vi "analoginput_software_trigger_daqmxbasemodified.vi"() -> ()   [LabVIEW 2014]
doc: "This VI compares analog data from a DAQ device in software to some trigger level. Once the condition is met the VI in software initiates a digital right to a pin on a DAQ device."
uses:
  <vilib>/_DAQmxBase/Internals/DAQmxBase Read (Analog 1D DBL NChan 1Samp).vi
  <vilib>/_DAQmxBase/Internals/DAQmxBase Timing (Sample Clock).vi
  <vilib>/_DAQmxBase/Internals/DAQmxBase Create Channel (AI-Voltage-Basic).vi
panel:
  in  "Analog Clock Source":tag
  in  "Analog Channel":tag="Dev1/ai0"
  in  "Analog Sample Mode":T1(ring)=enum."Hardware Timed Single Point"
  in  "Sample Rate":dbl=1000.0 format="%#_13g"
  in  "Trigger Level":dbl=2.0 format="%#_13g"
  in  "Trigger Type":T2(ring)
  out "Trigger?":bool
  out "Input Signal":dbl[](graph)
  in  "stop":bool
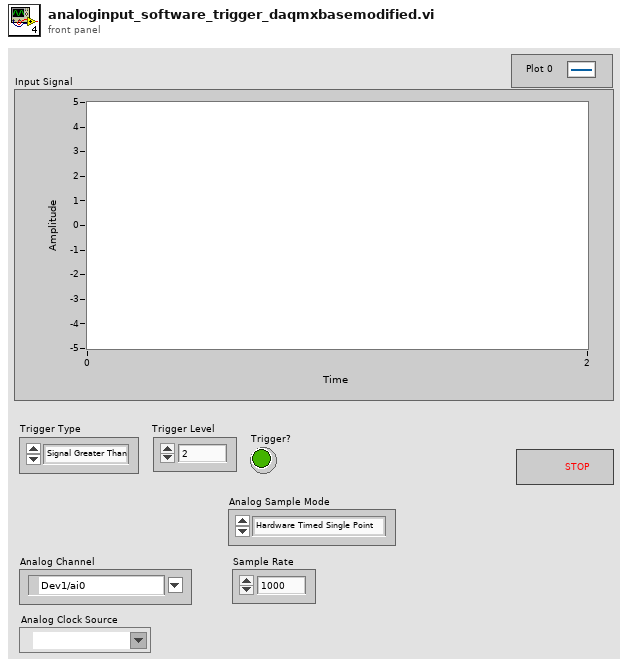
[diagram p1: front panel]
types:
  T1 = enum16{"Finite Samples", "Continuous Samples", "Hardware Timed Single Point"}
  T2 = enum16{"Signal Greater Than", "Signal Less Than", "Signal Equal To", "None"}
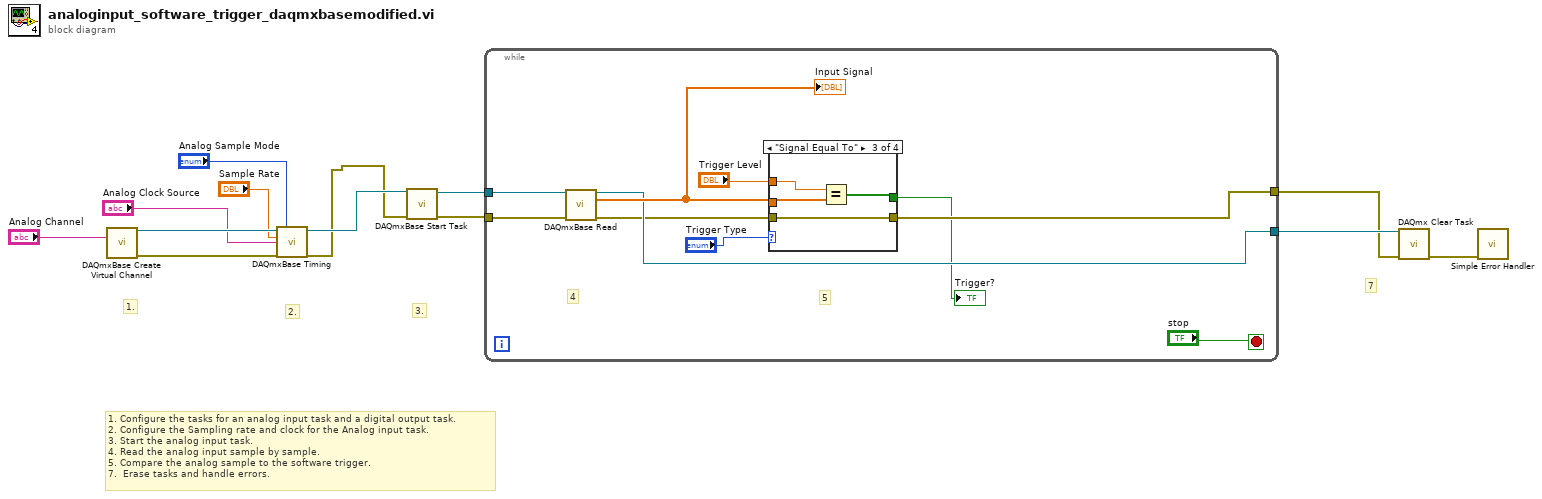
[diagram p0: block diagram]
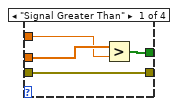
[diagram p2: hidden frame]
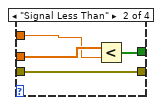
[diagram p3: hidden frame]
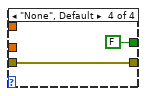
[diagram p4: hidden frame]
diagram:
  # "3."
  # "1. Configure the tasks for an analog input task and a digital output task. \n2. Configure the Sampling rate and clock for the Analog input task.\n3. Start the analog input task.\n4. Read the analog input sample by sample.\n5. Compare the analog sample to the software trigger.\n7.  Erase tasks and handle errors."
  # "7"
  # "2."
  # "1."
  n1 = call-poly <vilib>:"DAQmxBase Create Virtual Channel.vi"("physical channels"="Analog Channel") -> ("task out"=w13:refnum<k21>, "error out"=w12:errorcluster)  [unwired: 13 in]
  n2 = call-poly <vilib>:"DAQmxBase Timing.vi"("task/channels in"=w13, "sample mode"="Analog Sample Mode", "rate"="Sample Rate", "source"="Analog Clock Source", "error in"=w12) -> ("task out"=w11:refnum<k21>, "error out"=w1:errorcluster)  [unwired: 9 in]
  n3 = call <vilib>:"DAQmxBase Start Task.vi"("task/channels in"=w11, "error in"=w1) -> ("task out"=w10:refnum<k21>, "error out"=w9:errorcluster)  [unwired: 12 in]
  n4 = while {
    tunnel: w10 -> [w23]
    tunnel: w9 -> [w22]
    tunnel: [w15] -> w2
    tunnel: [w19] -> w6
    stop <- "stop" stop-if-true
    # "5"
    # "4"
    n5 = call-poly <vilib>:"DAQmxBase Read.vi"("task/channels in"=w23, "error in"=w22) -> ("task out"=w19:refnum<k21>, "data"=w21:dbl[], "error out"=w18:errorcluster)  [unwired: 11 in]
    "Input Signal" <- w21
    n6 = case shown="\"Signal Equal To\"" "Trigger Type" {
      tunnel: w21 -> [w27 w30 w35 _]
      tunnel: [w26 w31 w34 _] -> _
      tunnel: w18 -> [w25 w29 w33 w37]
      tunnel: [w25 w29 w33 w37] -> w15
      tunnel: "Trigger Level" -> [w24 w28 w32 _]
      tunnel: [_ _ _ FALSE] -> w14
      frame "Signal Greater Than" {
        n7 = Greater?(x=w27, y=w24) -> (0:w26:bool[])
      }
      frame "Signal Less Than" {
        n8 = Less?(x=w30, y=w28) -> (x < y?=w31:bool[])
      }
      frame "Signal Equal To" {
        n9 = Equal?(x=w32, y=w35) -> (x = y?=w34:bool[])
      }
      frame "None", Default {
      }
    }
    "Trigger?" <- w14
  }
  n10 = call "DAQmx Clear Task.vi"("task in"=w6, "error in"=w2) -> ("error out"=w5:errorcluster)  [unwired: 13 in]
  n11 = call <vilib>:"Simple Error Handler.vi"("error in (no error)"=w5) -> ()  [unwired: 4 in, 5 out]
